vi "Write_CubeLiftOutput.vi"(8 "error in (no error)":errorcluster, 10 "CubeLiftOutput":T1 {"LiftControlMode" items=["PercentOutput"=0, "Position"=1, "Velocity"=2, "Current"=3, "Follower"=5, "MotionProfile"=6, "MotionMagic"=7, "MotionMagicArc"=8, "MotionProfileArc"=10, "Disabled"=15]}, 11 "CubeLiftData in":refnum<class "CubeLiftData.lvclass">) -> (0 "error out":errorcluster, 3 "CubeLiftData out":refnum<class "CubeLiftData.lvclass">)   [LabVIEW 2017, in "CubeLiftData.lvclass"]
uses:
  CubeLiftData.lvclass
  Team-code/CubeLiftOutput.ctl
  <vilib>/Rock Robotics/WPI/ThirdParty/Phoenix-LabVIEW/Motor Controller/Controls/CTRE_Phoenix_MotorControl_ControlMode.ctl
  CubeLiftData.lvclass/CubeLiftData.ctl
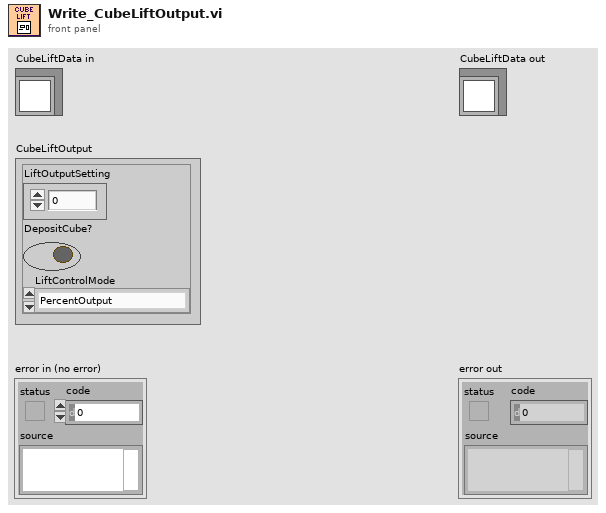
[diagram p1: front panel]
types:
  T1 = typedef "CubeLiftData.lvclass/CubeLiftOutput.ctl" = cluster{"LiftOutputSetting":dbl, "DepositCube?":bool, "LiftControlMode":T2}
  T2 = typedef "CTRE_Phoenix_MotorControl_ControlMode.ctl" = u16
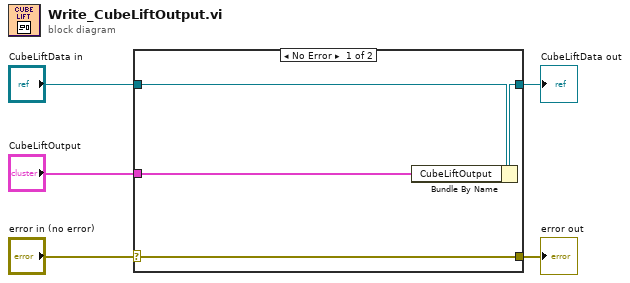
[diagram p0: block diagram]
diagram:
  n1 = case shown="No Error" "error in (no error)" {
    selector: "error in (no error)" -> [w9 w10]
    tunnel: [w9 w10] -> w4
    tunnel: [w7 w11] -> w2
    tunnel: "CubeLiftData in" -> [w8 w11]
    tunnel: "CubeLiftOutput" -> [w6 _]
    frame No Error {
      n2 = Bundle By Name(cluster=w8, "CubeLiftOutput"=w6) -> (w7:refnum<class "CubeLiftData.lvclass">)
    }
    frame Error {
    }
  }
  "error out" <- w4
  "CubeLiftData out" <- w2
